vi "GUI_v2.vi"() -> ()   [LabVIEW 2023]
uses:
  Serial - Settings.ctl
  <vilib>/Utility/miscctls.llb/LV3DPointTypeDef.ctl
  <vilib>/Utility/miscctls.llb/LVRGBAColorTypeDef.ctl
  e2109eba-4716-5941-afb7-b0faa504542a.vi
  327bca25-9371-1e41-8126-f95c64e27f6d.vi
  <vilib>/Analysis/coordinate.llb/3D Cartesian Coordinate Rotation (Euler) (Array).vi
  abf5b892-6ba6-6f43-be19-45be42e399fc.vi
  <vilib>/Array/Sort 2D Array - Pop Stack.vi
  <vilib>/Array/Sort 2D Array - Push Stack.vi
  327bca25-9371-1e41-8126-f95c64e27f6d.vi/269d4b3b-47f5-49e3-8884-44851e4dd9d5.vi
  327bca25-9371-1e41-8126-f95c64e27f6d.vi/6d99389c-673d-4efb-bf33-19b32bcf4cf8.vi
  abf5b892-6ba6-6f43-be19-45be42e399fc.vi/269d4b3b-47f5-49e3-8884-44851e4dd9d5.vi
  abf5b892-6ba6-6f43-be19-45be42e399fc.vi/6d99389c-673d-4efb-bf33-19b32bcf4cf8.vi
  <vilib>/Instr/_visa.llb/VISA Configure Serial Port (Instr).vi
  <vilib>/picture/3D Picture Control/Object/Create Object (drawable).vi
  <vilib>/picture/3D Picture Control/Object/Add Object (no reference).vi
  <vilib>/picture/3D Picture Control/NI_3D Picture Control.lvlib
  <vilib>/Analysis/NI_AALPro.lvlib
panel:
  out "Serial Settings:Number of Bytes at Serial Port":u32
  in  "Serial Settings":T1={"baud rate"=115200, "data bits"=8, "parity"=enum."None", "stop bits"=10, "flow control"=0} {"flow control" items=["None"=0, "XON/XOFF"=1, "RTS/CTS"=2, "DTR/DSR"=4]; "stop bits" items=["1.0"=10, "1.5"=15, "2.0"=20]; "data bits" min=5 max=8 step=1; "baud rate" items=["75"=75, "110"=110, "134"=134, "150"=150, "300"=300, "600"=600, "1200"=1200, "1800"=1800, "2400"=2400, "4800"=4800, "7200"=7200, "9600"=9600, "14400"=14400, "19200"=19200, "28800"=28800, "38400"=38400, "56000"=56000, "57600"=57600, "115200"=115200, "128000"=128000, "230400"=230400]}
  out "concatenated string":string
  out "length":i32
  in  "Draw Mode":T2(ring)
  in  "Front":bool
  out "3D Picture":refnum<vi>(3d-picture)
  out "Number of Points":i32
  in  "Clear":bool
  in  "From File?":bool
  in  "File path":path
  out "Input Coordinates":string
  out "Read Buffer":string
  in  "VISA resource name":refnum<visa-resource-name>
  in  "Rotation":cluster{"Roll":i32, "Pitch":i32, "Yaw":i32} {"Yaw" scale=0.0..180.0; "Pitch" scale=0.0..180.0; "Roll" scale=0.0..5.0}
  in  "Back":bool
  in  "Up":bool
  in  "Down":bool
  in  "Right":bool
  in  "Sphere":bool
  in  "Cube":bool
  in  "Left":bool
  in  "[ESC]":bool
  # "1. Connect to ESP32 via serial VISA\n2. Select model\n3. Play around!"
  # "X"
  # "Y"
  # "Z"
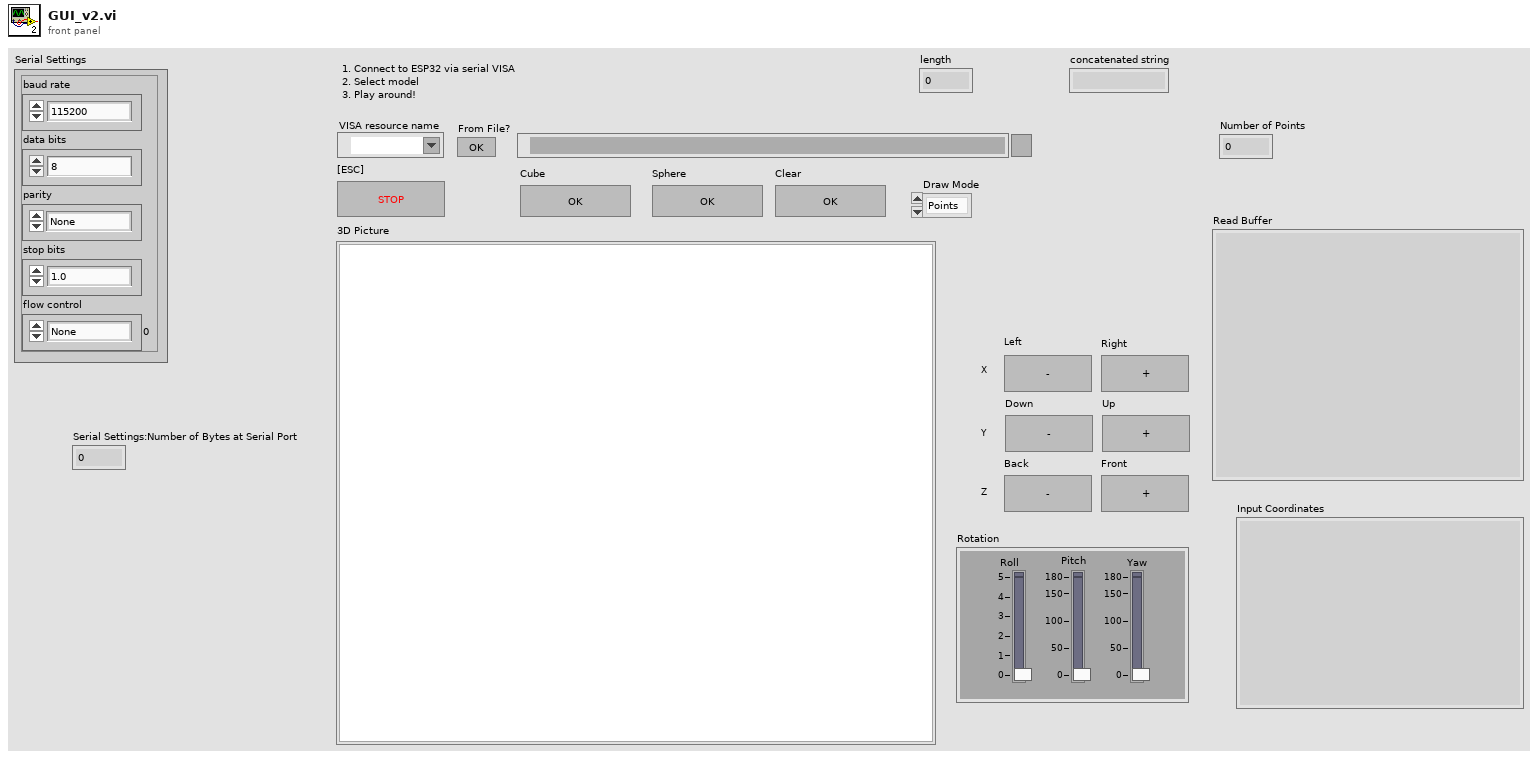
[diagram p1: front panel]
types:
  T1 = typedef "Serial - Settings.ctl" = cluster{"baud rate":u32, "data bits":u16, "parity":enum16{"None", "Odd", "Even", "Mark", "Space"}, "stop bits":u16, "flow control":u16}
  T2 = enum16{"Points", "Lines", "Line Strip", "Line Loop", "Triangles", "Triangle Strip", "Triangle Fan", "Quads", "Quad Strip", "Polygon"}
  T3 = enum16{"Inherit Value", "No Culling", "Cull Back Face", "Cull Front Face", "Cull Both Faces"}
  T4 = enum16{"Inherit Value", "Counterclockwise", "Clockwise"}
  T5 = enum16{"Inherit Value", "Points", "Wireframe", "Polygons"}
  T6 = cluster{"Red":sgl, "Green":sgl, "Blue":sgl, "Alpha":sgl}
  T7 = typedef "LVRGBAColorTypeDef.ctl" = cluster{"Red":sgl, "Green":sgl, "Blue":sgl, "Alpha":sgl}
  T8 = enum16{"Overall", "Per Primitive", "Per Vertex", "Binding Off"}
  T9 = typedef "LV3DPointTypeDef.ctl" = cluster{"X":sgl, "Y":sgl, "Z":sgl}
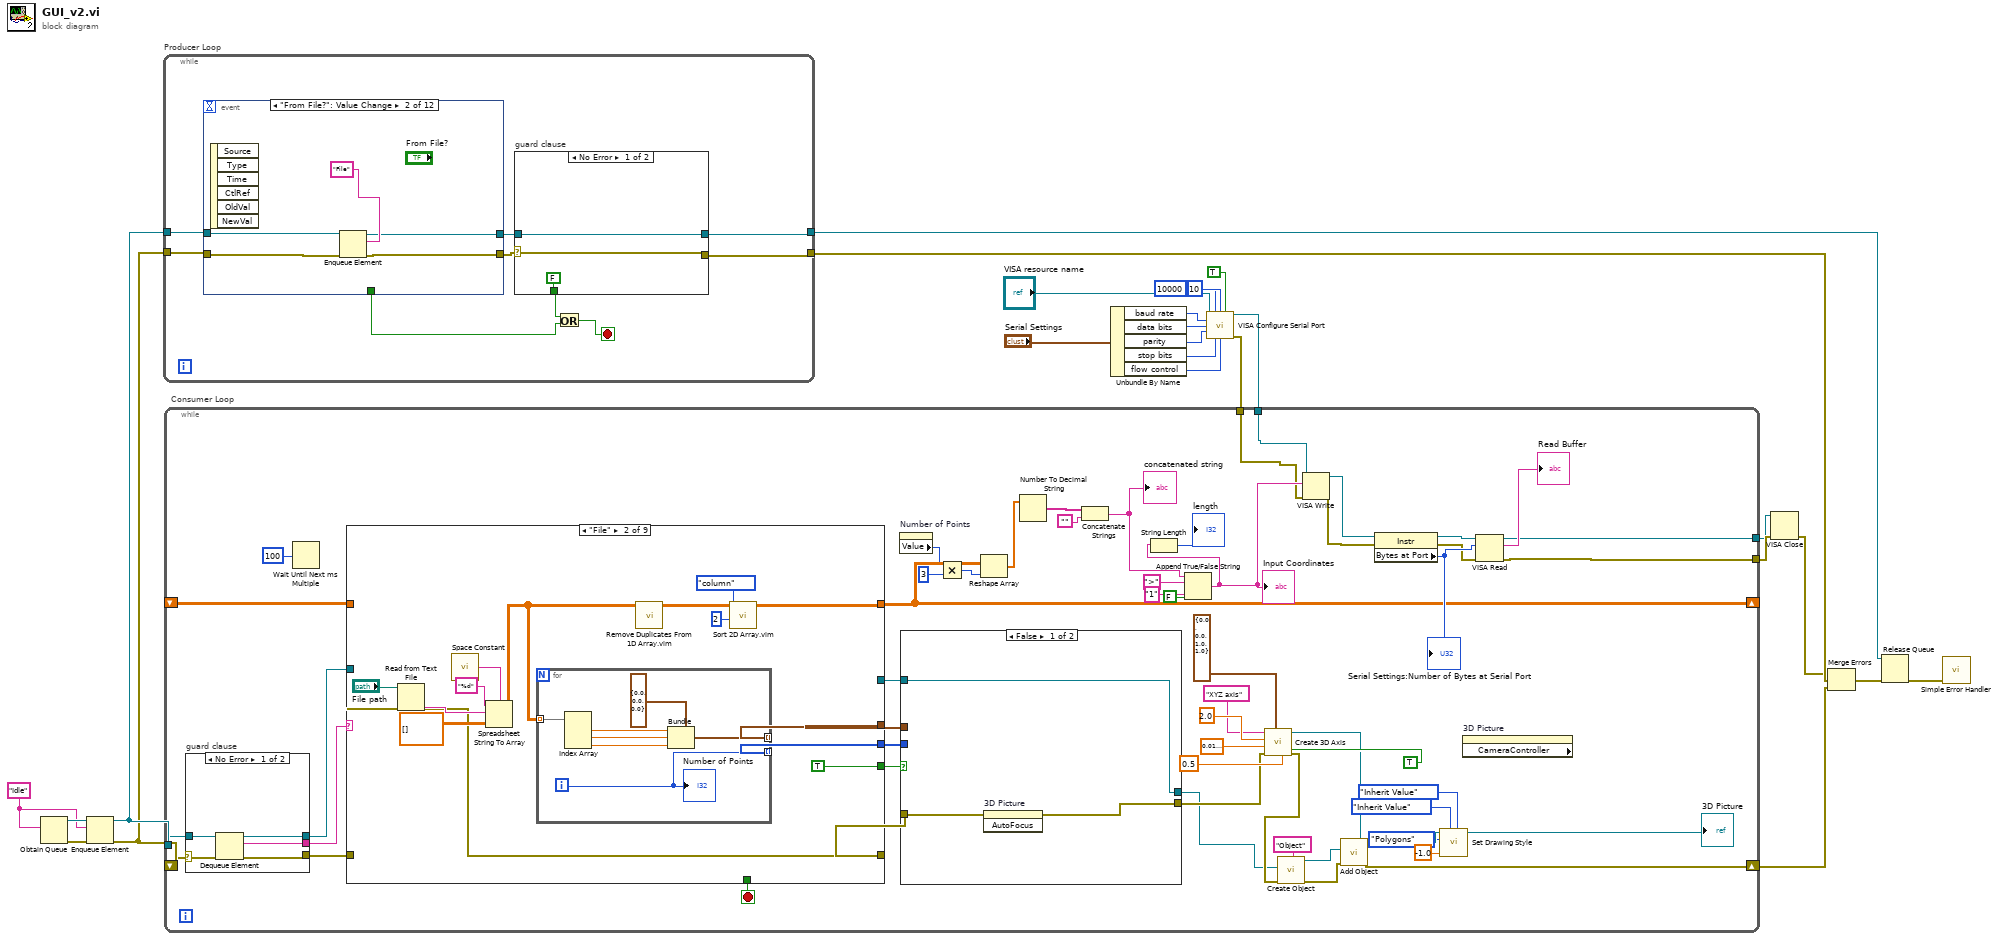
[diagram p0: block diagram]
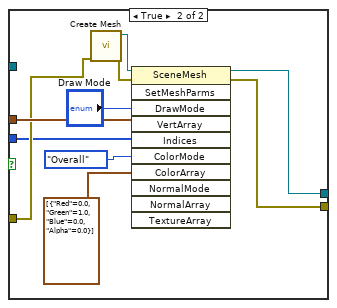
[diagram p2: hidden frame]
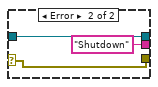
[diagram p3: hidden frame]
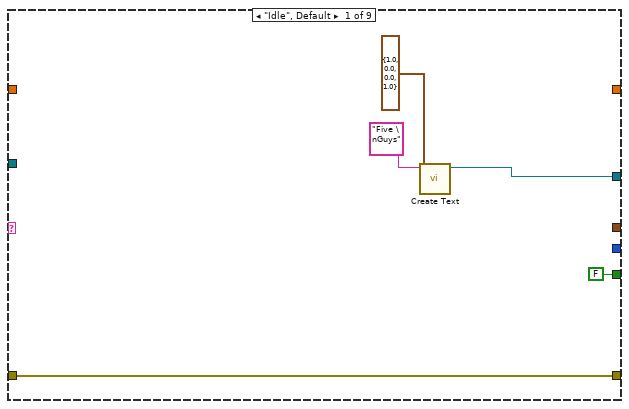
[diagram p4: hidden frame]
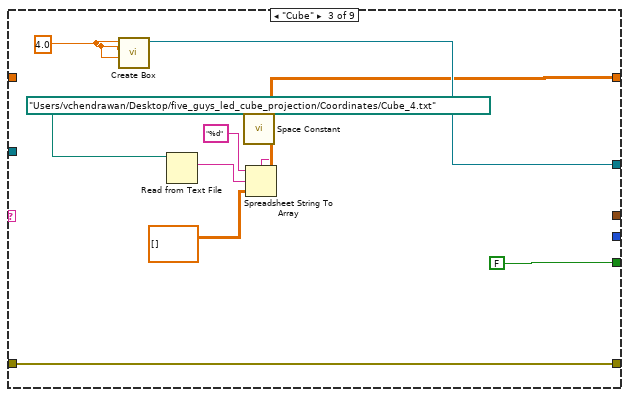
[diagram p5: hidden frame]
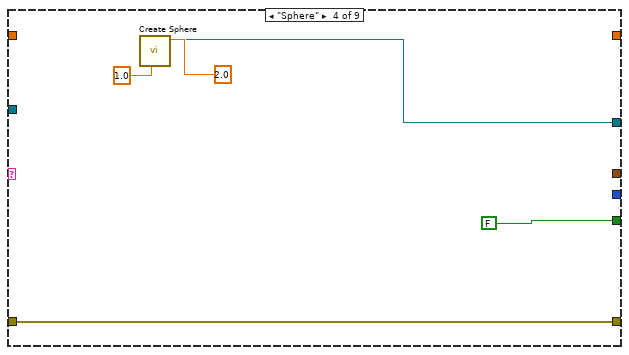
[diagram p6: hidden frame]
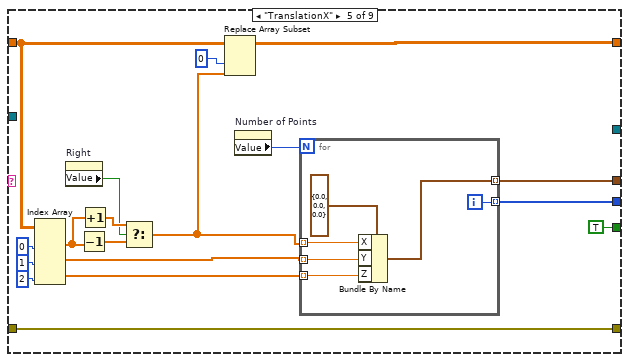
[diagram p7: hidden frame]
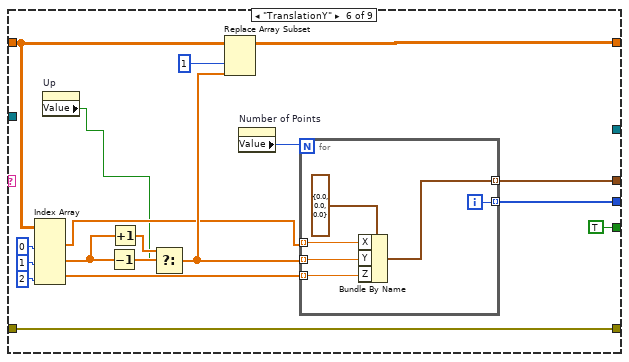
[diagram p8: hidden frame]
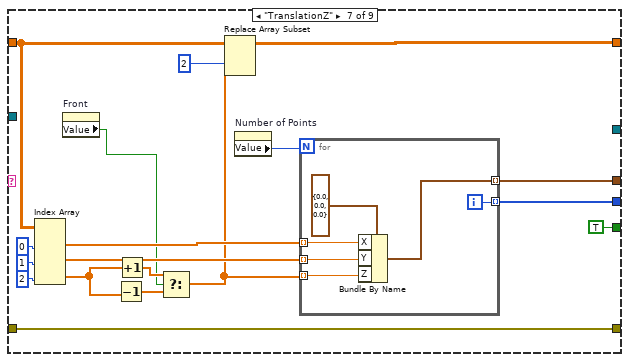
[diagram p9: hidden frame]
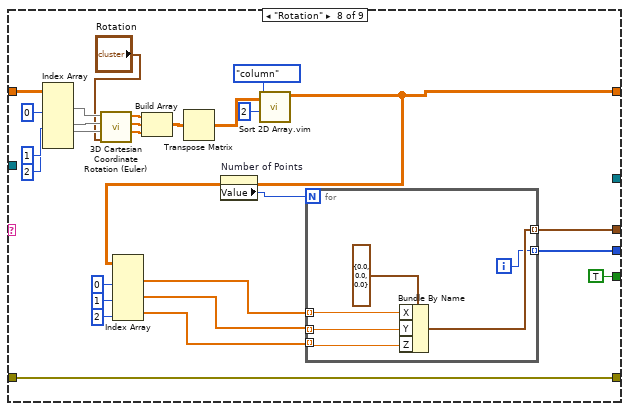
[diagram p10: hidden frame]
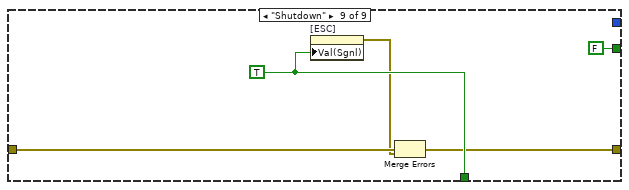
[diagram p11: hidden frame]
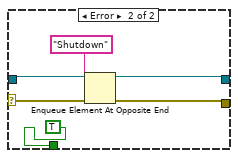
[diagram p12: hidden frame]
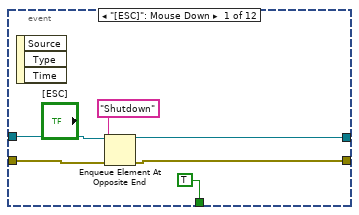
[diagram p13: hidden frame]
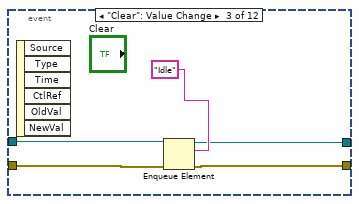
[diagram p14: hidden frame]
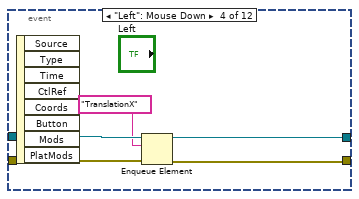
[diagram p15: hidden frame]
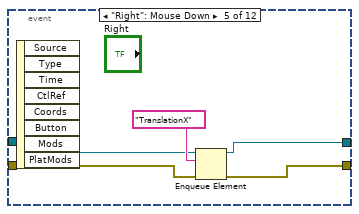
[diagram p16: hidden frame]
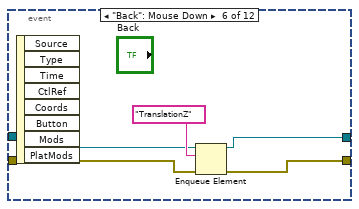
[diagram p17: hidden frame]
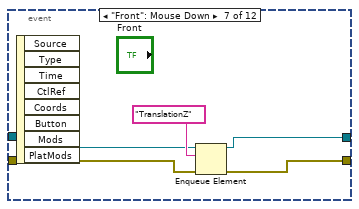
[diagram p18: hidden frame]
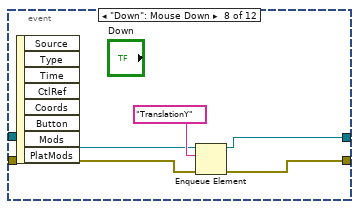
[diagram p19: hidden frame]
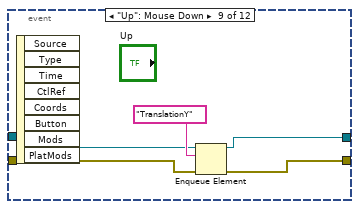
[diagram p20: hidden frame]
diagram:
  w23 = "Idle"
  n1 = Obtain Queue(element data type=w23) -> (queue out=w24:refnum<queue>, error out=w25:errorcluster)  [unwired: 4 in, 1 out]
  n2 = Enqueue Element(queue=w24, element=w23, error in (no error)=w25) -> (queue out=w22:refnum<queue>, error out=w21:errorcluster)  [unwired: 1 in, 1 out]
  n3 = while "Producer Loop" {
    tunnel: [w27] -> w18
    tunnel: [w26] -> w20
    tunnel: w22 -> [w31]
    tunnel: w21 -> [w30]
    stop <- w32 stop-if-true
    n4 = event shown="[1] \"From File?\": Value Change" {
      selector: _ -> [_ _ _ _ _ _ _ _ _ _ _ _]
      dyn-events: _ -> [_ _ _ _ _ _ _ _ _ _ _ _]
      timeout: _ -> [_ _ _ _ _ _ _ _ _ _ _ _]
      tunnel: [TRUE _ _ _ _ _ _ _ _ _ _ _] -> w34
      tunnel: [w47 w50 w55 w60 w65 w70 w75 w80 w85 w90 w95 w103] -> w28
      tunnel: [w46 w51 w56 w63 w66 w71 w76 w81 w86 w91 w96 w102] -> w29
      tunnel: w31 -> [w45 w52 w57 w64 w68 w73 w78 w83 w88 w93 w98 w101]
      tunnel: w30 -> [w44 w53 w58 w62 w67 w72 w77 w82 w87 w92 w97 w100]
      event "[ESC]": Mouse Down {
        n5 = event-data() -> ()  [unwired: 1 in, 3 out]
        n6 = Enqueue Element At Opposite End(queue=w45, element="Shutdown", error in (no error)=w44) -> (queue out=w46:refnum<queue>, error out=w47:errorcluster)  [unwired: 1 in, 1 out]
      }
      event "From File?": Value Change {
        n7 = event-data() -> ()  [unwired: 1 in, 6 out]
        n8 = Enqueue Element(queue=w52, element="File", error in (no error)=w53) -> (queue out=w51:refnum<queue>, error out=w50:errorcluster)  [unwired: 1 in, 1 out]
      }
      event "Clear": Value Change {
        n9 = event-data() -> ()  [unwired: 1 in, 6 out]
        n10 = Enqueue Element(queue=w57, element="Idle", error in (no error)=w58) -> (queue out=w56:refnum<queue>, error out=w55:errorcluster)  [unwired: 1 in, 1 out]
      }
      event "Left": Mouse Down {
        n11 = event-data() -> ()  [unwired: 1 in, 8 out]
        n12 = Enqueue Element(queue=w64, element="TranslationX", error in (no error)=w62) -> (queue out=w63:refnum<queue>, error out=w60:errorcluster)  [unwired: 1 in, 1 out]
      }
      event "Right": Mouse Down {
        n13 = event-data() -> ()  [unwired: 1 in, 8 out]
        n14 = Enqueue Element(queue=w68, element="TranslationX", error in (no error)=w67) -> (queue out=w66:refnum<queue>, error out=w65:errorcluster)  [unwired: 1 in, 1 out]
      }
      event "Back": Mouse Down {
        n15 = event-data() -> ()  [unwired: 1 in, 8 out]
        n16 = Enqueue Element(queue=w73, element="TranslationZ", error in (no error)=w72) -> (queue out=w71:refnum<queue>, error out=w70:errorcluster)  [unwired: 1 in, 1 out]
      }
      event "Front": Mouse Down {
        n17 = event-data() -> ()  [unwired: 1 in, 8 out]
        n18 = Enqueue Element(queue=w78, element="TranslationZ", error in (no error)=w77) -> (queue out=w76:refnum<queue>, error out=w75:errorcluster)  [unwired: 1 in, 1 out]
      }
      event "Down": Mouse Down {
        n19 = event-data() -> ()  [unwired: 1 in, 8 out]
        n20 = Enqueue Element(queue=w83, element="TranslationY", error in (no error)=w82) -> (queue out=w81:refnum<queue>, error out=w80:errorcluster)  [unwired: 1 in, 1 out]
      }
      event "Up": Mouse Down {
        n21 = event-data() -> ()  [unwired: 1 in, 8 out]
        n22 = Enqueue Element(queue=w88, element="TranslationY", error in (no error)=w87) -> (queue out=w86:refnum<queue>, error out=w85:errorcluster)  [unwired: 1 in, 1 out]
      }
      event "Cube": Value Change {
        n23 = event-data() -> ()  [unwired: 1 in, 6 out]
        n24 = Enqueue Element(queue=w93, element="Cube", error in (no error)=w92) -> (queue out=w91:refnum<queue>, error out=w90:errorcluster)  [unwired: 1 in, 1 out]
      }
      event "Sphere": Value Change {
        n25 = event-data() -> ()  [unwired: 1 in, 6 out]
        n26 = Enqueue Element(queue=w98, element="Sphere", error in (no error)=w97) -> (queue out=w96:refnum<queue>, error out=w95:errorcluster)  [unwired: 1 in, 1 out]
      }
      event "Rotation": Value Change {
        n27 = event-data() -> ()  [unwired: 1 in, 1 out]
        n28 = Enqueue Element(queue=w101, element="Rotation", error in (no error)=w100) -> (queue out=w102:refnum<queue>, error out=w103:errorcluster)  [unwired: 1 in, 1 out]
      }
    }
    n29 = case "guard clause" shown="No Error" w28 {
      selector: w28 -> [w36 w41]
      tunnel: w29 -> [w37 w42]
      tunnel: [w37 w39] -> w27
      tunnel: [w36 w40] -> w26
      tunnel: [FALSE TRUE] -> w33
      frame No Error {
      }
      frame Error {
        n30 = Enqueue Element At Opposite End(queue=w42, element="Shutdown", error in (no error)=w41) -> (queue out=w39:refnum<queue>, error out=w40:errorcluster)  [unwired: 1 in, 1 out]
      }
    }
    n31 = Or(x=w33, y=w34) -> (x .or. y?=w32:bool)
  }
  n32 = Unbundle By Name("Serial Settings") -> ("baud rate"=w10:u32, "data bits"=w9:u16, "parity"=w8:enum16{"None", "Odd", "Even", "Mark", "Space"}, "stop bits"=w7:u16, "flow control"=w6:u16)
  n33 = call-poly "VISA Configure Serial Port"("VISA resource name"="VISA resource name", "timeout (10sec)"=u32 10000, "termination char\n(0xA = '\\n' = LF)"=u8 10 ("termination char\n(0xA = '\\n' = LF)"), "Enable Termination\nChar (T)"=TRUE ("Enable Termination\nChar (T)"), "baud rate (9600)"=w10, "data bits (8)"=w9, "parity (0:none)"=w8, "stop bits (10: 1 bit)"=w7, "flow control (0:none)"=w6) -> ("VISA resource name out"=w2:refnum<visa-resource-name>, "error out"=w3:errorcluster)  [unwired: 5 in]
  n34 = while "Consumer Loop" {
    tunnel: w22 -> [w160]
    shift-right: [w121] -> w17
    shift-left: w21 -> [w157]
    shift-right: [w119] -> _
    shift-left: _ -> [w151]
    tunnel: w2 -> [w105]
    tunnel: w3 -> [w106]
    tunnel: [w137] -> w15
    tunnel: [w136] -> w14
    stop <- w158 stop-if-true
    n35 = case "guard clause" shown="No Error" w157 {
      selector: w157 -> [w177 w180]
      tunnel: w160 -> [w178 w181]
      tunnel: [w176 w180] -> w159
      tunnel: [w175 "Shutdown"] -> w134
      tunnel: [w174 w181] -> w135
      frame No Error {
        n36 = Dequeue Element(queue=w178, error in (no error)=w177) -> (queue out=w174:refnum<queue>, element=w175:string, error out=w176:errorcluster)  [unwired: 1 in, 1 out]
      }
      frame Error {
      }
    }
    n37 = Wait Until Next ms Multiple(millisecond multiple=u32 100) -> ()  [unwired: 1 out]
    n38 = case shown="\"File\"" w134 {
      tunnel: w159 -> [w186 w193 w218 w220 w240 w264 w288 w322 w332]
      tunnel: w135 -> [_ _ _ _ _ _ _ _ _]
      tunnel: [_ _ _ _ _ _ _ _ w333] -> w158
      tunnel: [w186 w192 w218 w220 w240 w264 w288 w322 w330] -> w150
      tunnel: [_ w200 _ _ w235 w257 w281 w299 _] -> w155
      tunnel: [_ w199 _ _ w234 w256 w280 w298 _] -> w154
      tunnel: [w184 _ w217 w222 _ _ _ _ _] -> w153
      tunnel: [FALSE TRUE FALSE FALSE TRUE TRUE TRUE TRUE FALSE] -> w152
      tunnel: [_ w189 w213 _ w228 w263 w287 w306 _] -> w119
      tunnel: w151 -> [_ _ _ _ w239 w262 w286 w318 _]
      frame "Idle", Default {
        n39 = call <vilib>:"Create Text.vi"("Color"=T6 {"Red"=1.0, "Green"=0.0, "Blue"=0.0, "Alpha"=1.0}, "Text"="Five \nGuys") -> ("New Text Refnum"=w184:refnum<vi>)  [unwired: 8 in, 1 out]
      }
      frame "File" {
        n40 = Read from Text File(file (use dialog)="File path", error in=w193) -> (text=w197:string, error out=w192:errorcluster)  [unwired: 2 in, 2 out]
        n41 = call <vilib>:"Space Constant.vi"() -> ("String"=w196:string)
        n42 = Spreadsheet String To Array(delimiter (Tab)=w196, format string="%d", spreadsheet string=w197, array type (2D Dbl)=sgl[][] []) -> (array=w191:sgl[][])
        n43 = for {
          tunnel: w191 -> [w202] mode=indexing
          tunnel: [w204] -> w200 mode=indexing
          tunnel: [w203] -> w199 mode=indexing
          i -> [w203]
          n44 = Index Array(array=w202) -> (element #1=w207:sgl, element #2=w206:sgl, element #3=w205:sgl)  [unwired: 3 in]
          n45 = Bundle(cluster=T9 {"X"=0.0, "Y"=0.0, "Z"=0.0} ("3D Point"), "X"=w207, "Y"=w206, "Z"=w205) -> (w204:T9)
          "Number of Points" <- w203
        }
        n46 = call "Remove Duplicates From 1D Array.vim"("array"=w191) -> ("array with duplicates removed"=w190:sgl[][])  [unwired: 10 in]
        n47 = call "Sort 2D Array.vim"("index"=2, "dimension to index (column)"=enum16{"column", "row"}."column", "2D array"=w190) -> ("sorted 2D array"=w189:sgl[][])  [unwired: 7 in, 1 out]
      }
      frame "Cube" {
        w209 = 4.0
        n48 = call <vilib>:"Create Box.vi"("Length Z"=w209, "Length Y"=w209, "Length X"=w209) -> ("New Box Refnum"=w217:refnum<vi>)  [unwired: 7 in, 1 out]
        n49 = Read from Text File(file (use dialog)=path "/Users/vchendrawan/Desktop/five_guys_led_cube_projection/Coordinates/Cube_4.txt") -> (text=w214:string)  [unwired: 3 in, 3 out]
        n50 = call <vilib>:"Space Constant.vi"() -> ("String"=w211:string)
        n51 = Spreadsheet String To Array(delimiter (Tab)=w211, format string="%d", spreadsheet string=w214, array type (2D Dbl)=sgl[][] []) -> (array=w213:sgl[][])
      }
      frame "Sphere" {
        n52 = call <vilib>:"Create Sphere.vi"("Detail"=sgl 1.0, "Radius"=sgl 2.0) -> ("New Sphere Refnum"=w222:refnum<vi>)  [unwired: 8 in, 1 out]
      }
      frame "TranslationX" {
        n53 = Index Array "Index Array"(array=w239, index (col) #1=0 ("disabled index (col)"), index (col) #2=1 ("index (col)"), index (col) #3=2 ("index (col)")) -> (element #1=w232:dbl[], element #2=w225:dbl[], element #3=w224:dbl[])  [unwired: 3 in]
        n54 = property on="Right" class="Bool (strict)"() -> ("Value"=w230:bool)  [unwired: 2 in, 2 out]
        n55 = Decrement(x=w232) -> (x-1=w233:dbl[])
        n56 = Increment(x=w232) -> (x+1=w231:dbl[])
        n57 = Select(t=w231, s=w230, f=w233) -> (s? t:f=w226:dbl[])
        n58 = Replace Array Subset(array=w239, new element=w226, index (col)=0 ("disabled index (col)")) -> (w228:dbl[][])  [unwired: 1 in]
        n59 = property on="Number of Points" class="DigNum (strict)"() -> ("Value"=w229:i32)  [unwired: 2 in, 2 out]
        n60 = for {
          N: w229 -> [_]
          tunnel: w226 -> [w247] mode=indexing
          tunnel: w225 -> [w246] mode=indexing
          tunnel: w224 -> [w245] mode=indexing
          tunnel: [w244] -> w235 mode=indexing
          tunnel: [w242] -> w234 mode=indexing
          i -> [w242]
          n61 = Bundle By Name(cluster=T9 {"X"=0.0, "Y"=0.0, "Z"=0.0} ("3D Point"), "X"=w247, "Y"=w246, "Z"=w245) -> (w244:T9)
        }
      }
      frame "TranslationY" {
        n62 = Index Array "Index Array"(array=w262, index (col) #1=0 ("disabled index (col)"), index (col) #2=1 ("index (col)"), index (col) #3=2 ("index (col)")) -> (element #1=w251:dbl[], element #2=w253:dbl[], element #3=w258:dbl[])  [unwired: 3 in]
        n63 = property on="Up" class="Bool (strict)"() -> ("Value"=w250:bool)  [unwired: 2 in, 2 out]
        n64 = Decrement(x=w253) -> (x-1=w255:dbl[])
        n65 = Increment(x=w253) -> (x+1=w254:dbl[])
        n66 = Select(t=w254, s=w250, f=w255) -> (s? t:f=w252:dbl[])
        n67 = Replace Array Subset(array=w262, new element=w252, index (col)=1 ("disabled index (col)")) -> (w263:dbl[][])  [unwired: 1 in]
        n68 = property on="Number of Points" class="DigNum (strict)"() -> ("Value"=w249:i32)  [unwired: 2 in, 2 out]
        n69 = for {
          N: w249 -> [_]
          tunnel: w251 -> [w271] mode=indexing
          tunnel: w252 -> [w270] mode=indexing
          tunnel: w258 -> [w269] mode=indexing
          tunnel: [w268] -> w257 mode=indexing
          tunnel: [w266] -> w256 mode=indexing
          i -> [w266]
          n70 = Bundle By Name(cluster=T9 {"X"=0.0, "Y"=0.0, "Z"=0.0} ("3D Point"), "X"=w271, "Y"=w270, "Z"=w269) -> (w268:T9)
        }
      }
      frame "TranslationZ" {
        n71 = Index Array "Index Array"(array=w286, index (col) #1=0 ("disabled index (col)"), index (col) #2=1 ("index (col)"), index (col) #3=2 ("index (col)")) -> (element #1=w276:dbl[], element #2=w282:dbl[], element #3=w277:dbl[])  [unwired: 3 in]
        n72 = property on="Front" class="Bool (strict)"() -> ("Value"=w272:bool)  [unwired: 2 in, 2 out]
        n73 = Decrement(x=w277) -> (x-1=w279:dbl[])
        n74 = Increment(x=w277) -> (x+1=w278:dbl[])
        n75 = Select(t=w278, s=w272, f=w279) -> (s? t:f=w275:dbl[])
        n76 = Replace Array Subset(array=w286, new element=w275, index (col)=2 ("disabled index (col)")) -> (w287:dbl[][])  [unwired: 1 in]
        n77 = property on="Number of Points" class="DigNum (strict)"() -> ("Value"=w274:i32)  [unwired: 2 in, 2 out]
        n78 = for {
          N: w274 -> [_]
          tunnel: w276 -> [w295] mode=indexing
          tunnel: w282 -> [w294] mode=indexing
          tunnel: w275 -> [w293] mode=indexing
          tunnel: [w292] -> w281 mode=indexing
          tunnel: [w290] -> w280 mode=indexing
          i -> [w290]
          n79 = Bundle By Name(cluster=T9 {"X"=0.0, "Y"=0.0, "Z"=0.0} ("3D Point"), "X"=w295, "Y"=w294, "Z"=w293) -> (w292:T9)
        }
      }
      frame "Rotation" {
        n80 = Index Array "Index Array"(array=w318, index (col) #1=0 ("disabled index (col)"), index (col) #2=1 ("index (col)"), index (col) #3=2 ("index (col)")) -> (element #1=w317:dbl[], element #2=w316:dbl[], element #3=w315:dbl[])  [unwired: 3 in]
        n81 = call-poly <vilib>:"3D Cartesian Coordinate Rotation (Euler).vi"("Euler Angles"="Rotation", "Z"=w315, "Y"=w316, "X"=w317) -> ("Z Out"=w312:dbl[], "Y Out"=w313:dbl[], "X Out"=w314:dbl[])  [unwired: 4 in, 1 out]
        n82 = Build Array(w314, w313, w312) -> (w311:dbl[][])
        n83 = Transpose Matrix(1:w311) -> (0:w308:dbl[][])
        n84 = property on="Number of Points" class="DigNum (strict)"() -> ("Value"=w297:i32)  [unwired: 2 in, 2 out]
        n85 = call "Sort 2D Array.vim"("index"=2, "dimension to index (column)"=enum16{"column", "row"}."column", "2D array"=w308) -> ("sorted 2D array"=w306:dbl[][])  [unwired: 7 in, 1 out]
        n86 = Index Array "Index Array"(array=w306, index (col) #1=0 ("disabled index (col)"), index (col) #2=1 ("index (col)"), index (col) #3=2 ("index (col)")) -> (element #1=w302:dbl[], element #2=w301:dbl[], element #3=w300:dbl[])  [unwired: 3 in]
        n87 = for {
          N: w297 -> [_]
          tunnel: w302 -> [w327] mode=indexing
          tunnel: w301 -> [w326] mode=indexing
          tunnel: w300 -> [w325] mode=indexing
          tunnel: [w324] -> w299 mode=indexing
          tunnel: [w323] -> w298 mode=indexing
          i -> [w323]
          n88 = Bundle By Name(cluster=T9 {"X"=0.0, "Y"=0.0, "Z"=0.0} ("3D Point"), "X"=w327, "Y"=w326, "Z"=w325) -> (w324:T9)
        }
      }
      frame "Shutdown" {
        w333 = TRUE
        n89 = property on="[ESC]" class="Bool (strict)"("Val(Sgnl)"=w333) -> (error out=w331:errorcluster)  [unwired: 2 in, 1 out]
        n90 = Merge Errors(w332, w331) -> (w330:errorcluster)
      }
    }
    n91 = property on="Number of Points" class="DigNum (strict)"() -> ("Value"=w116:i32)  [unwired: 2 in, 2 out]
    n92 = case shown="False" w152 {
      tunnel: w155 -> [_ w170]
      tunnel: w154 -> [_ w166]
      tunnel: w153 -> [w163 _]
      tunnel: w150 -> [w162 w169]
      tunnel: [w161 w168] -> w131
      tunnel: [w163 w167] -> w129
      frame False {
        n93 = invoke on="3D Picture" class="SceneGraphDisp (strict)" method="AutoFocus"(error in=w162) -> (error out=w161:errorcluster)  [unwired: 2 in, 2 out]
      }
      frame True {
        n94 = call <vilib>:"Create Mesh.vi"("error in (no error)"=w169) -> ("error out"=w173:errorcluster, "New Mesh Refnum"=w172:refnum<vi>)  [unwired: 9 in]
        n95 = invoke class="SceneMesh" method="SetMeshParms"(reference=w172, error in=w173, "DrawMode"="Draw Mode", "VertArray"=w170, "Indices"=w166, "ColorMode"=T8."Overall" ("Color Binding Mode"), "ColorArray"=T7[] [{"Red"=0.0, "Green"=1.0, "Blue"=0.0, "Alpha"=0.0}] ("Color Array")) -> (reference out=w167:refnum<vi>, error out=w168:errorcluster)  [unwired: 4 in, 9 out]
      }
    }
    n96 = Multiply(x=w116, y=3) -> (x*y=w118:i32)
    n97 = Reshape Array(w119, w118) -> (w110:dbl[])
    n98 = Number To Decimal String(number=w110) -> (decimal integer string=w108:string[])  [unwired: 1 in]
    n99 = Concatenate Strings(w108, "") -> (w107:string)
    "concatenated string" <- w107
    n100 = Append True/False String(1:FALSE ("selector"), 2:"1" ("false string"), 3:">" ("true string"), 4:w107) -> (0:w111:string)
    "Input Coordinates" <- w111
    n101 = String Length(string=w111) -> (length=→"length":i32)
    n102 = call <vilib>:"Create 3D Axis.vi"("Character Size"=sgl 0.5, "Axis label?"=TRUE, "Color"=T6 {"Red"=0.0, "Green"=0.0, "Blue"=1.0, "Alpha"=1.0}, "error in (no error)"=w131, "Radius"=sgl 0.02, "Length"=sgl 2.0, "Name"="XYZ axis") -> ("error out"=w130:errorcluster, "New Object Refnum"=w132:refnum<vi>)  [unwired: 3 in]
    n103 = call-poly <vilib>:"Create Object.vi"("error in (no error)"=w130, "Geometry"=w129, "Name"="Object") -> ("error out"=w127:errorcluster, "Scene:New Object"=w128:refnum<vi>)  [unwired: 7 in]
    n104 = VISA Write(VISA resource name=w105, write buffer=w111, error in (no error)=w106) -> (VISA resource name out=w139:refnum<visa-resource-name>, error out=w141:errorcluster)  [unwired: 1 out]
    n105 = call-poly <vilib>:"Add Object.vi"("error in (no error)"=w127, "New Object In"=w128, "Scene Object In"=w132) -> ("error out"=w121:errorcluster, "Scene Object Out"=w126:refnum<vi>)  [unwired: 7 in]
    n106 = property on="Property Node" class="Instr"(reference=w139, error in=w141) -> (reference out=w140:refnum<visa-resource-name>, error out=w142:errorcluster, "Bytes at Port"=w143:u32)
    "Serial Settings:Number of Bytes at Serial Port" <- w143
    n107 = call <vilib>:"Set Drawing Style.vi"("Face Culling Mode"=T3."Inherit Value", "Frontface Mode"=T4."Inherit Value", "Size"=-1.0, "Mode"=T5."Polygons", "Scene Object In"=w126) -> ("Scene Object Out"=→"3D Picture":refnum<vi>)  [unwired: 5 in, 1 out]
    n108 = property on="3D Picture" class="SceneGraphDisp (strict)" props=["CameraController"]() -> ()  [unwired: 2 in, 3 out]
    n109 = VISA Read(VISA resource name=w140, byte count=w143, error in (no error)=w142) -> (VISA resource name out=w136:refnum<visa-resource-name>, read buffer=→"Read Buffer":string, error out=w137:errorcluster)  [unwired: 1 out]
  }
  n110 = VISA Close(VISA resource name=w14, error in (no error)=w15) -> (error out=w13:errorcluster)
  n111 = Merge Errors(w13, w20, w17) -> (w19:errorcluster)
  n112 = Release Queue(queue=w18, error in (no error)=w19) -> (error out=w12:errorcluster)  [unwired: 1 in, 2 out]
  n113 = call <vilib>:"Simple Error Handler.vi"("error in (no error)"=w12) -> ()  [unwired: 4 in, 5 out]
